vi "ParseMsgFirmwareVersion.vi"(8 "error in":errorcluster, 11 "Sysex Message":u8[](array[numeric]) format="%x") -> (0 "error out":errorcluster, 1 "IsValidReply":bool, 3 "FirmataFirmwareVersion":string)   [LabVIEW 2020, in "FirmataClient.lvlib"]
doc: "Parse a message according to the Firmata Protocol Requirements. \n- https://github.com/firmata/protocol\n- https://github.com/firmata/protocol/blob/master/protocol.md"
uses:
  FirmataClient.lvlib
  controls/FirmataProtocolConstants.ctl
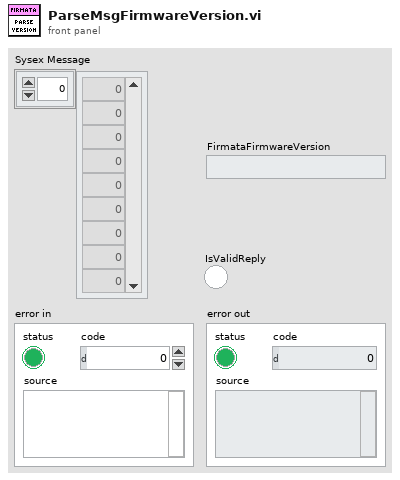
[diagram p1: front panel]
types:
  T1 = typedef "FirmataClient.lvlib/FirmataProtocolConstants.ctl" = u16
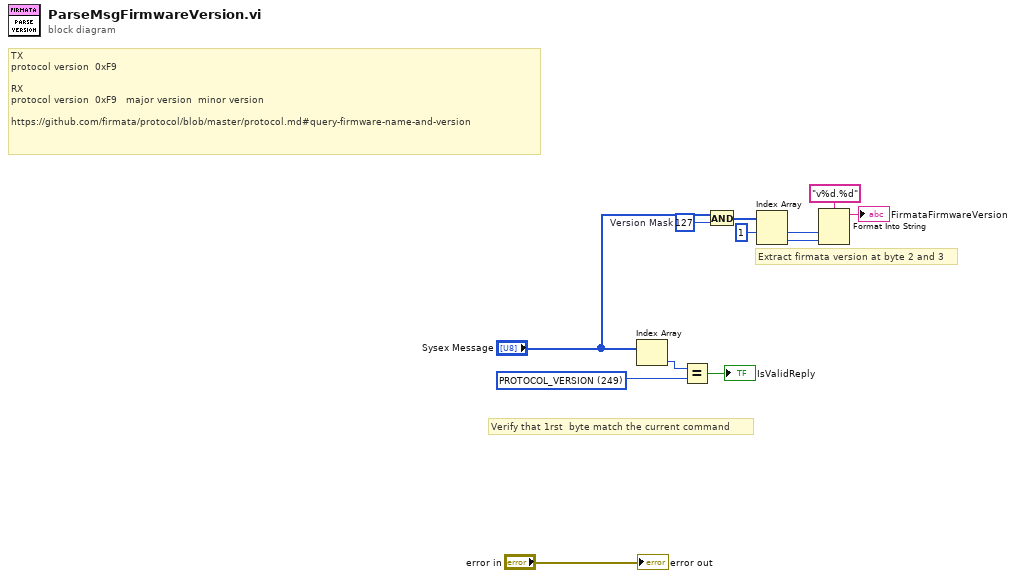
[diagram p0: block diagram]
diagram:
  w1 = T1 249 items=["ANALOG_IO_MESSAGE"=224, "DIGITAL_IO_MESSAGE"=144, "REPORT_ANALOG_PIN"=192, "REPORT_DIGITAL_PORT"=208, "START_SYSEX"=240, "END_SYSEX"=247, "SET_PIN_MODE"=244, "SET_DIGITAL_PIN_VALUE"=245, "PROTOCOL_VERSION"=249, "SYSTEM_RESET"=255, "SYSEX.EXTENDED_ID"=0, "SYSEX.RESERVED_USER_COMMANDs"=1, "SYSEX.ANALOG_MAPPING_QUERY"=105, "SYSEX.ANALOG_MAPPING_RESPONSE"=106, "SYSEX.CAPABILITY_QUERY"=107, "SYSEX.CAPABILITY_RESPONSE"=108, "SYSEX.PIN_STATE_QUERY"=109, "SYSEX.PIN_STATE_RESPONSE"=110, "SYSEX.REPORT_FIRMWARE"=121, "SYSEX.EXTENDED_ANALOG"=111, "SYSEX.STRING_DATA"=113, "SYSEX.REALTIME"=127, "SYSEX.NON_REALTIME"=126, "SYSEX.SAMPLING_INTERVAL"=122] ("FimataProtocolConstants")
  w6 = u8 127  # Version Mask
  # "Extract firmata version at byte 2 and 3"
  # "Verify that 1rst  byte match the current command"
  # "TX\nprotocol version \t0xF9 \t\t\n\nRX\nprotocol version \t0xF9 \t\tmajor version \tminor version\n\nhttps://github.com/firmata/protocol/blob/master/protocol.md#query-firmware-name-and-version"
  n1 = Index Array(array="Sysex Message") -> (element=w2:u8)  [unwired: 1 in]
  n2 = Equal?(x=w2, y=w1) -> (x = y?=→"IsValidReply":bool)
  n3 = And(x="Sysex Message", y=w6) -> (x .and. y?=w5:u8[])
  n4 = Index Array(array=w5, index #1=1 ("index")) -> (element #1=w10:u8, element #2=w9:u8)  [unwired: 1 in]
  n5 = Format Into String(format string="v%d.%d", w10, w9) -> (resulting string=→"FirmataFirmwareVersion":string)  [unwired: 2 in, 1 out]
  "error out" <- "error in"
